vi "FindLowestInvaders.vi"(11 "InvaderPosArray_IN":T3) -> (0 "LowestRowIndexes":i32[](array[numeric]), 3 "LowestPositions":T1(array[cluster]))   [LabVIEW 2019]
uses:
  InvaderPositionArray.ctl
  move_dir_lr.ctl
panel:
  in  "InvaderPosArray":T2(array[cluster])
  in  "InvaderAlive":bool[][](array[boolean])
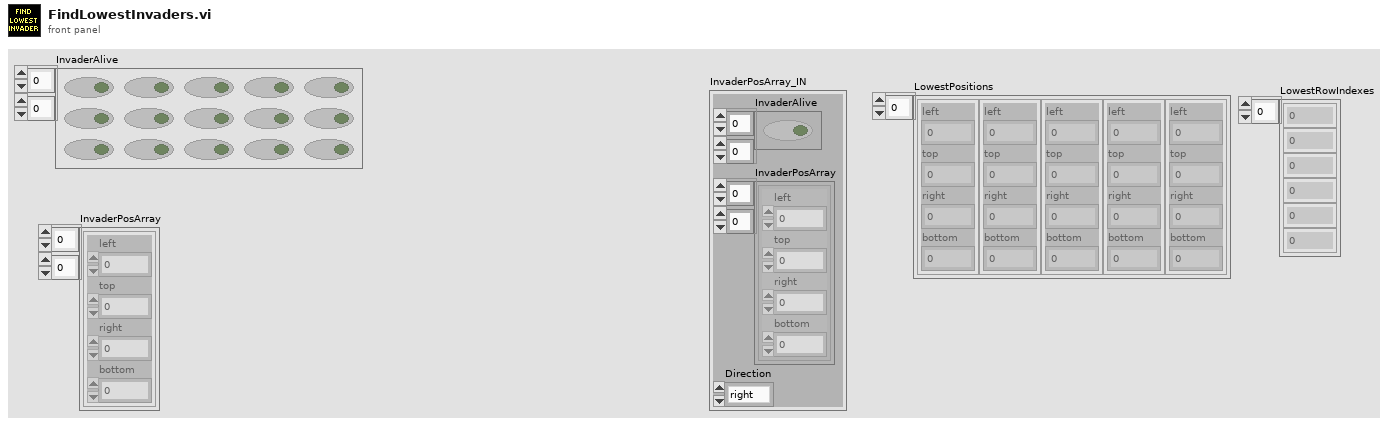
[diagram p1: front panel]
types:
  T1 = cluster{"left":i16, "top":i16, "right":i16, "bottom":i16}[]
  T2 = cluster{"left":i16, "top":i16, "right":i16, "bottom":i16}[][]
  T3 = typedef "InvaderPositionArray.ctl" = cluster{"InvaderAlive":bool[][], "InvaderPosArray":cluster{"left":i16, "top":i16, "right":i16, "bottom":i16}[][], "Direction":T4}
  T4 = typedef "move_dir_lr.ctl" = enum16{"right", "left"}
  T5 = cluster{"left":i16, "top":i16, "right":i16, "bottom":i16}
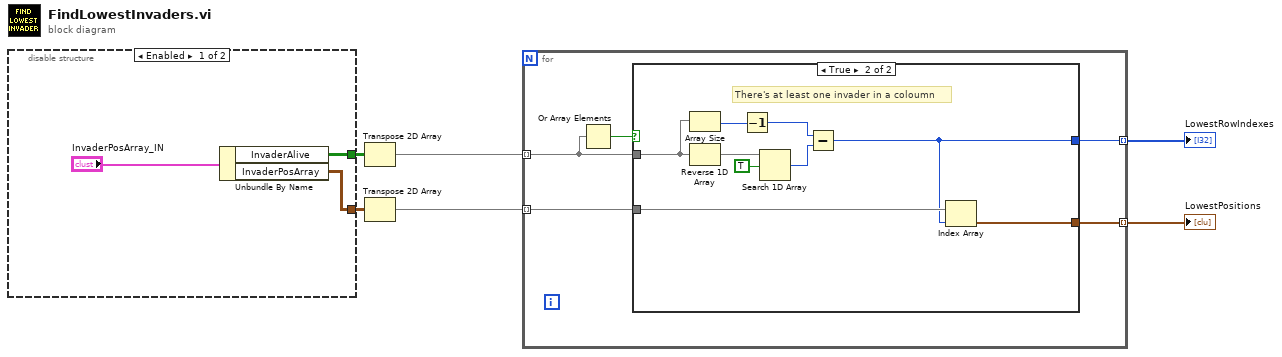
[diagram p0: block diagram]
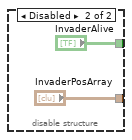
[diagram p2: hidden frame]
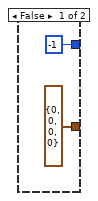
[diagram p3: hidden frame]
diagram:
  n1 = disable-structure shown="Enabled" {
    disable-tunnel: [w9 "InvaderAlive"] -> w6
    disable-tunnel: [w8 "InvaderPosArray"] -> w5
    frame Enabled {
      n2 = Unbundle By Name("InvaderPosArray_IN") -> ("InvaderAlive"=w9:bool[][], "InvaderPosArray"=w8:T2)
    }
    frame Disabled {
    }
  }
  n3 = Transpose 2D Array(2D array=w6) -> (transposed array=w3:bool[][])
  n4 = Transpose 2D Array(2D array=w5) -> (transposed array=w4:T2)
  n5 = for {
    tunnel: w3 -> [w16] mode=indexing
    tunnel: w4 -> [w14] mode=indexing
    tunnel: [w13] -> w1 mode=indexing
    tunnel: [w12] -> w2 mode=indexing
    n6 = Or Array Elements(Boolean array=w16) -> (logical OR=w15:bool)
    n7 = case shown="True" w15 {
      tunnel: w16 -> [_ w25]
      tunnel: [-1 w20] -> w12
      tunnel: w14 -> [_ w21]
      tunnel: [T5 {"left"=0, "top"=0, "right"=0, "bottom"=0} ("Rectangle") w19] -> w13
      frame False {
      }
      frame True {
        # "There's at least one invader in a coloumn"
        n8 = Array Size(array=w25) -> (size(s)=w24:i32)
        n9 = Reverse 1D Array(array=w25) -> (reversed array=w27:bool[])
        n10 = Decrement(x=w24) -> (x-1=w23:i32)
        n11 = Search 1D Array(1D array=w27, element=TRUE ("logical OR")) -> (index of element=w22:i32)  [unwired: 1 in]
        n12 = Subtract(x=w23, y=w22) -> (x-y=w20:i32)
        n13 = Index Array(array=w21, index=w20) -> (element=w19:T5)
      }
    }
  }
  "LowestRowIndexes" <- w2
  "LowestPositions" <- w1
